vi "Update Tree Edit Control.vi"(8 "Data Type":T1 items=["Tree Parent"=-1, "Numeric"=0, "String"=1, "Boolean"=2, "Enum"=3], 10 "Value":string, 11 "UI Data in":refnum<class "Settings UI.lvclass">) -> (3 "UI Data out":refnum<class "Settings UI.lvclass">)   [LabVIEW 2020, in "Output Sequencer.lvlib" / "Settings UI.lvclass"]
uses:
  Settings UI.lvclass
  Types/Data Type.ctl
  Types/Data Type Enum.ctl
  <vilib>/Utility/miscctls.llb/LVSelectionTypeDef.ctl
  Settings UI.lvclass/Settings UI.ctl
  Output Sequencer/Globals/Global Strings.vi
  Output Sequencer/Output Sequencer.lvclass
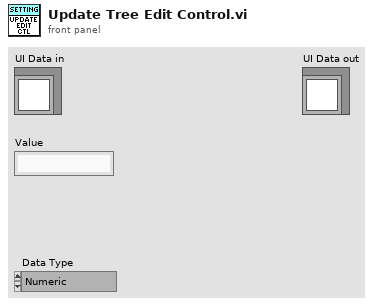
[diagram p1: front panel]
types:
  T1 = typedef "Output Sequencer.lvlib/Settings UI.lvclass/Data Type.ctl" = i16
  T2 = typedef "Output Sequencer.lvlib/Settings UI.lvclass/Data Type Enum.ctl" = enum16{"Numeric", "String", "Boolean", "Enum"}
  T3 = typedef "LVSelectionTypeDef.ctl" = cluster{"Selection Start":u32, "Selection End":u32}
  T4 = typedef "Output Sequencer.lvlib/Settings UI.lvclass/Tree Item Settings.ctl" = cluster{"Tree Label":string, "Indent Level":i32, "Data Type":T1, "Numeric Range":cluster{"Min":dbl, "Max":dbl, "Inc":dbl}, "Allowed Values":string[], "Default Value":string, "Description":string}
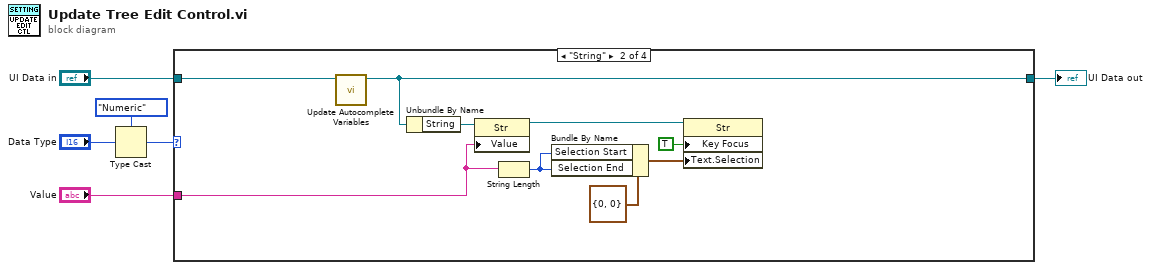
[diagram p0: block diagram]
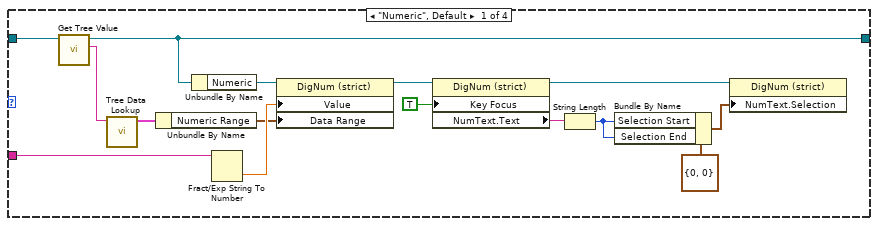
[diagram p2: hidden frame]
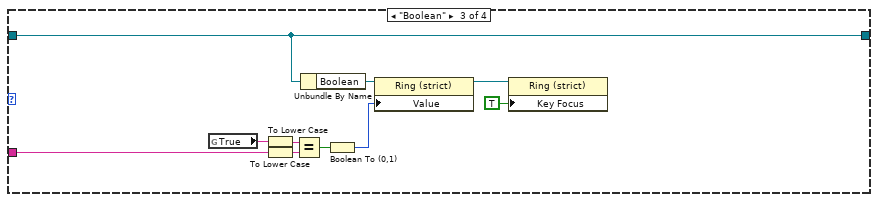
[diagram p3: hidden frame]
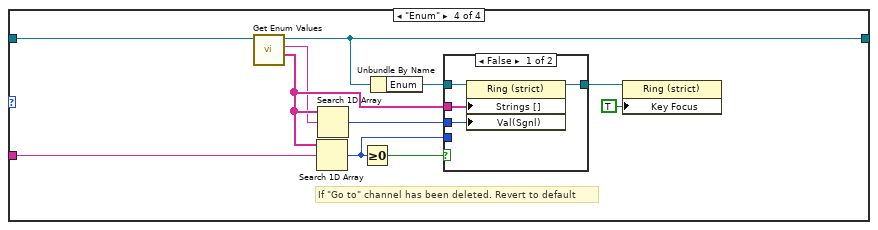
[diagram p4: hidden frame]
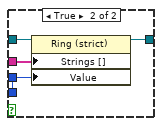
[diagram p5: hidden frame]
diagram:
  n1 = Type Cast(type=Data_Type_Enum."Numeric" ("Data Type"), x="Data Type") -> (*(type *) &x=w6:T2)
  n2 = case shown="\"String\"" w6 {
    tunnel: "UI Data in" -> [w8 w23 w31 w42]
    tunnel: "Value" -> [w21 w26 w40 w51]
    tunnel: [w7 w22 w31 w41] -> w3
    frame "Numeric", Default {
      n3 = call "Get Tree Value.vi"("UI Data in"=w8) -> ("Value"=w9:string, "UI Data out"=w7:refnum<class "Settings UI.lvclass">)  [unwired: 9 in]
      n4 = call "Tree Data Lookup.vi"("Tag in"=w9) -> ("Tree Data"=w10:T4)  [unwired: 5 in, 5 out]
      n5 = Unbundle By Name(w10) -> ("Numeric Range"=w11:cluster{"Min":dbl, "Max":dbl, "Inc":dbl})
      n6 = Unbundle By Name(w7) -> ("Numeric"=w14:refnum<vi>)
      n7 = Fract/Exp String To Number(string=w21) -> (number=w12:dbl)  [unwired: 3 in, 1 out]
      n8 = property class="DigNum (strict)"(reference=w14, "Value"=w12, "Data Range"=w11) -> (reference out=w13:refnum<vi>)  [unwired: 1 in, 1 out]
      n9 = property class="DigNum (strict)"(reference=w13, "Key Focus"=TRUE) -> (reference out=w20:refnum<vi>, "NumText.Text"=w19:string)  [unwired: 1 in, 1 out]
      n10 = String Length(string=w19) -> (length=w17:i32)
      n11 = Bundle By Name(cluster=T3 {"Selection Start"=0, "Selection End"=0} ("Numeric Text.Selection"), "Selection Start"=w17, "Selection End"=w17) -> (w16:T3)
      n12 = property class="DigNum (strict)"(reference=w20, "NumText.Selection"=w16) -> ()  [unwired: 1 in, 2 out]
    }
    frame "String" {
      n13 = call "Update Autocomplete Variables.vi"("UI Data in"=w23) -> ("UI Data out"=w22:refnum<class "Settings UI.lvclass">)  [unwired: 10 in]
      n14 = Unbundle By Name(w22) -> ("String"=w25:refnum<vi>)
      n15 = property class="Str"(reference=w25, "Value"=w26) -> (reference out=w24:refnum<vi>)  [unwired: 1 in, 1 out]
      n16 = String Length(string=w26) -> (length=w27:i32)
      n17 = Bundle By Name(cluster=T3 {"Selection Start"=0, "Selection End"=0} ("Text.Selection"), "Selection Start"=w27, "Selection End"=w27) -> (w28:T3)
      n18 = property class="Str"(reference=w24, "Key Focus"=TRUE, "Text.Selection"=w28) -> ()  [unwired: 1 in, 2 out]
    }
    frame "Boolean" {
      n19 = global read "Global Strings.vi" "True"() -> (w32:string)
      n20 = To Lower Case(string=w32) -> (all lower case string=w37:string)
      n21 = To Lower Case(string=w40) -> (all lower case string=w39:string)
      n22 = Equal?(x=w37, y=w39) -> (x = y?=w38:bool)
      n23 = Unbundle By Name(w31) -> ("Boolean"=w35:refnum<vi>)
      n24 = Boolean To (0,1)(Boolean=w38) -> (0, 1=w33:i16)
      n25 = property class="Ring (strict)"(reference=w35, "Value"=w33) -> (reference out=w34:refnum<vi>)  [unwired: 1 in, 1 out]
      n26 = property class="Ring (strict)"(reference=w34, "Key Focus"=TRUE) -> ()  [unwired: 1 in, 2 out]
    }
    frame "Enum" {
      # "If \"Go to\" channel has been deleted. Revert to default"
      n27 = call "Get Enum Values.vi"("UI Data in"=w42) -> ("Enum Values"=w47:string[], "Default Value"=w46:string, "UI Data out"=w41:refnum<class "Settings UI.lvclass">)  [unwired: 8 in]
      n28 = Search 1D Array(1D array=w47, element=w51) -> (index of element=w44:i32)  [unwired: 1 in]
      n29 = Search 1D Array(1D array=w47, element=w46) -> (index of element=w43:i32)  [unwired: 1 in]
      n30 = Greater Or Equal To 0?(x=w44) -> (x >= 0?=w45:bool)
      n31 = Unbundle By Name(w41) -> ("Enum"=w49:refnum<vi>)
      n32 = case shown="False" w45 {
        tunnel: w49 -> [w55 w59]
        tunnel: [w54 w58] -> w48
        tunnel: w47 -> [w53 w57]
        tunnel: w44 -> [_ w56]
        tunnel: w43 -> [w52 _]
        frame False {
          n33 = property class="Ring (strict)"(reference=w55, "Strings []"=w53, "Val(Sgnl)"=w52) -> (reference out=w54:refnum<vi>)  [unwired: 1 in, 1 out]
        }
        frame True {
          n34 = property class="Ring (strict)"(reference=w59, "Strings []"=w57, "Value"=w56) -> (reference out=w58:refnum<vi>)  [unwired: 1 in, 1 out]
        }
      }
      n35 = property class="Ring (strict)"(reference=w48, "Key Focus"=TRUE) -> ()  [unwired: 1 in, 2 out]
    }
  }
  "UI Data out" <- w3
